vi "read byte array.vi"(9 "specs":T1[](array[typedef]), 10 "elements":T4[](array[typedef]), 11 "byte array":u8[](array[numeric])) -> (0 "error out":errorcluster, 3 "message":variant)   [LabVIEW 2013, in "protocol buffers encoder.lvlib"]
uses:
  protocol buffers encoder.lvlib
  semiparse.ctl
  wire type.ctl
  message specification.ctl
  field descriptor.ctl
  quantity.ctl
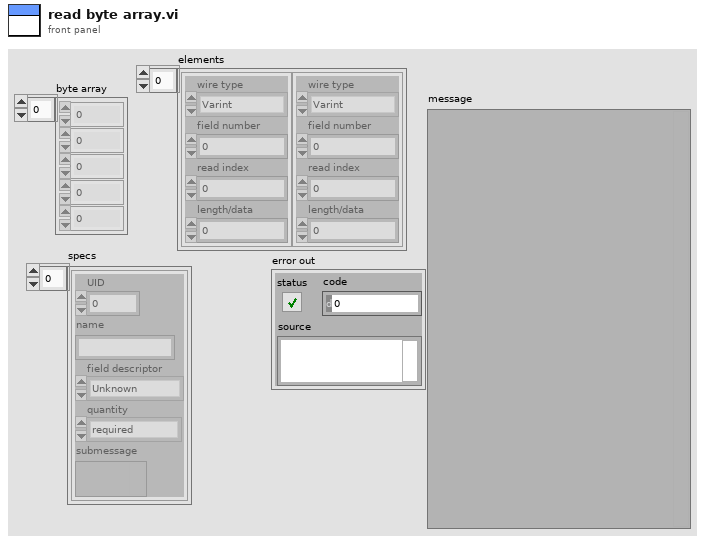
[diagram p1: front panel]
types:
  T1 = typedef "protocol buffers encoder.lvlib/message specification.ctl" = cluster{"UID":u64, "name":string, "field descriptor":T2, "quantity":T3, "submessage":variant}
  T2 = typedef "protocol buffers encoder.lvlib/field descriptor.ctl" = enum16{"Unknown", "dbl", "sgl", "i64", "u64", "i32", "fixed64", "fixed32", "bool", "string", "group", "message", "bytes", "u32", "enum", "sfixed32", "sfixed64", "sint32", "sint64"}
  T3 = typedef "protocol buffers encoder.lvlib/quantity.ctl" = enum16{"required", "optional", "repeated", "repeated/packed"}
  T4 = typedef "protocol buffers encoder.lvlib/semiparse.ctl" = cluster{"wire type":T5, "field number":u64, "read index":i32, "length/data":u64}
  T5 = typedef "protocol buffers encoder.lvlib/wire type.ctl" = enum8{"Varint", "64 bit", "Length Delimited", "Start Group", "End Group", "32 bit"}
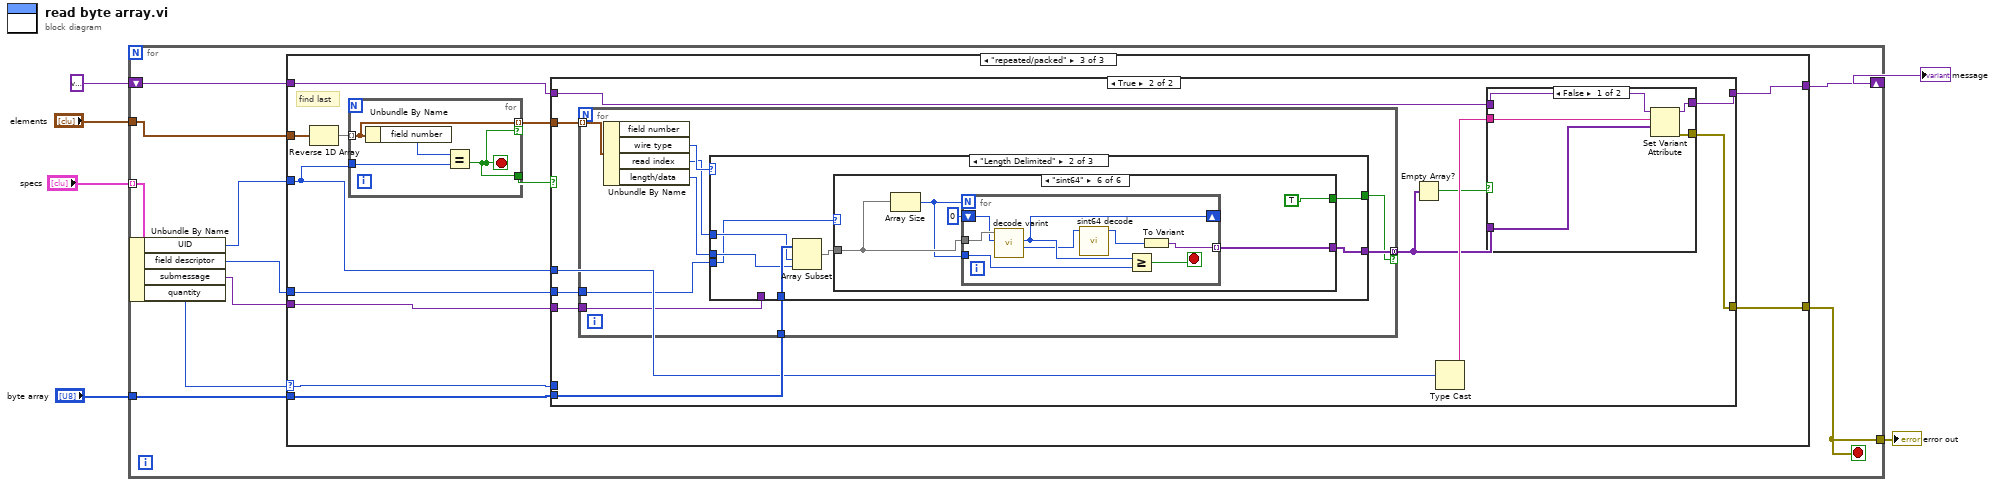
[diagram p0: block diagram]
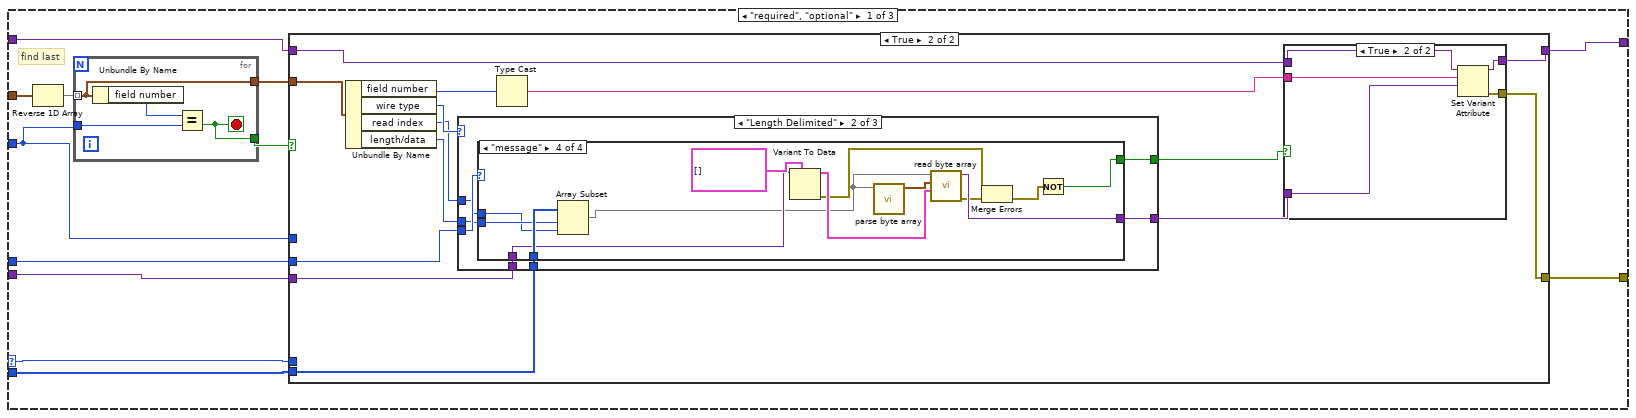
[diagram p2: hidden frame]
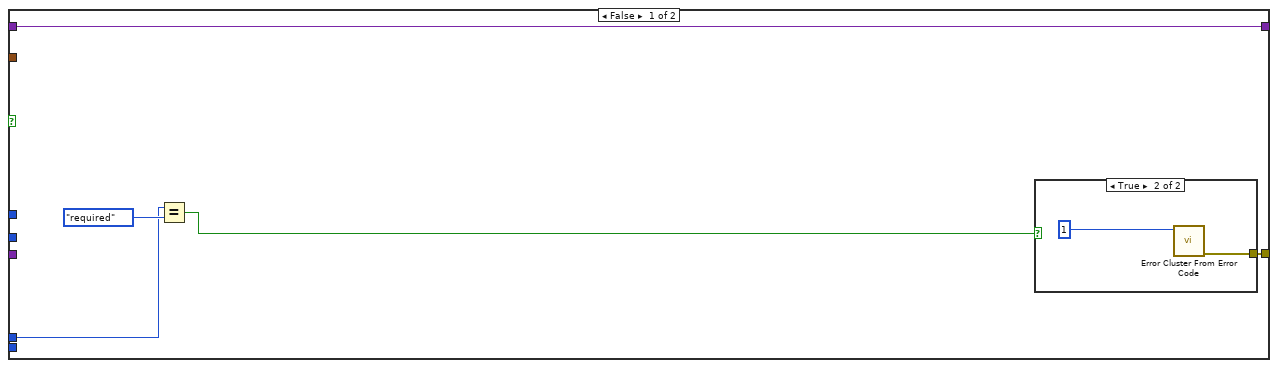
[diagram p3: hidden frame]
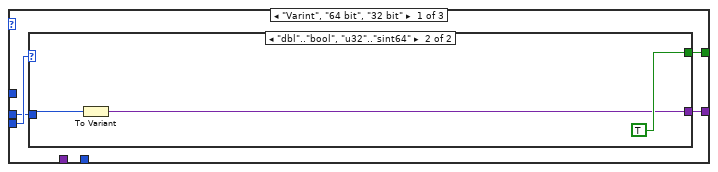
[diagram p5: hidden frame]
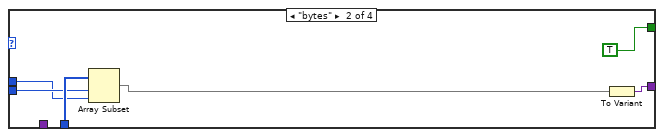
[diagram p8: hidden frame]
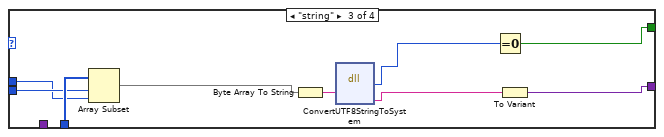
[diagram p9: hidden frame]
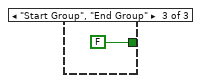
[diagram p10: hidden frame]
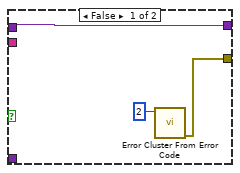
[diagram p11: hidden frame]
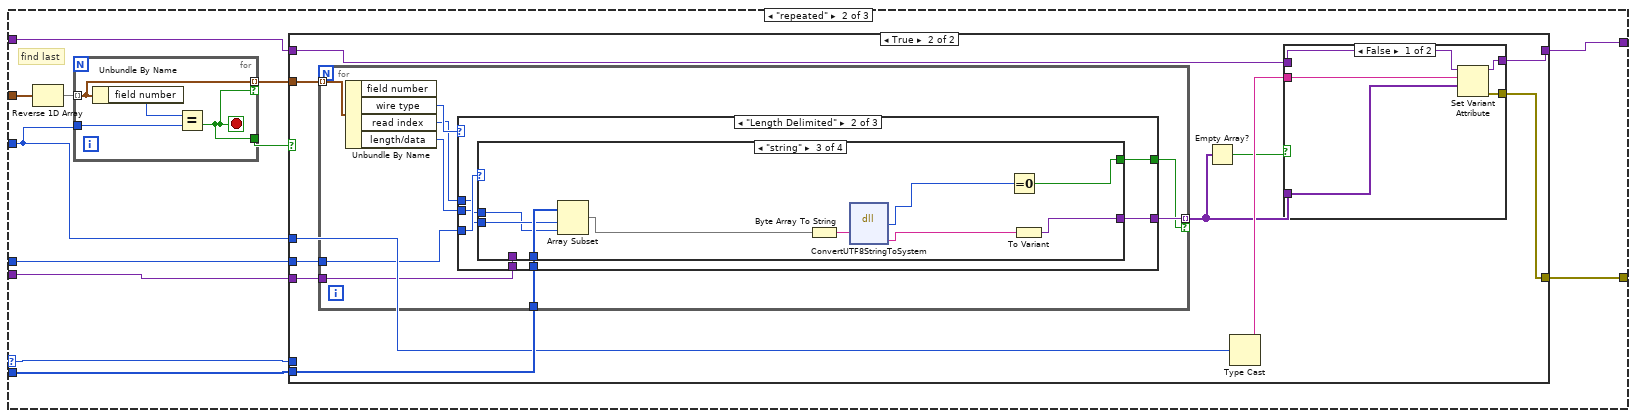
[diagram p12: hidden frame]
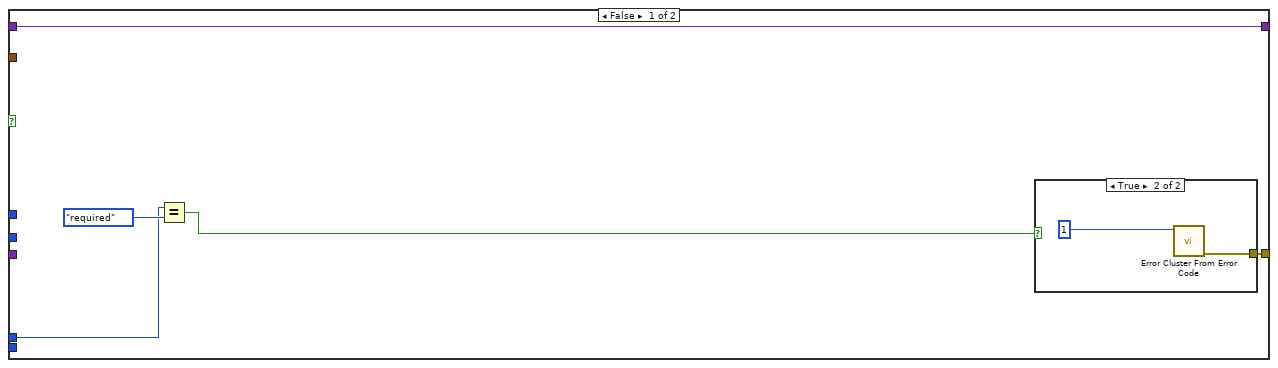
[diagram p13: hidden frame]
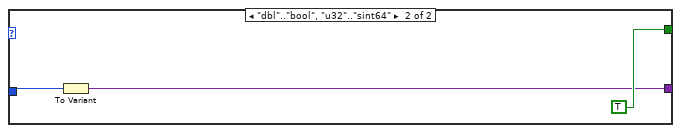
[diagram p16: hidden frame]
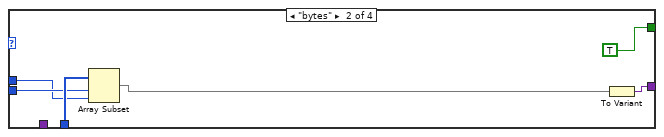
[diagram p18: hidden frame]
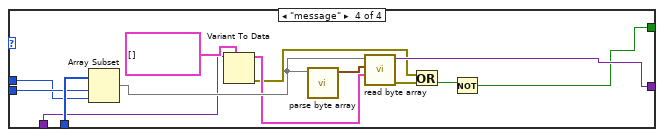
[diagram p19: hidden frame]
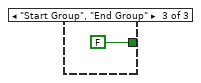
[diagram p20: hidden frame]
diagram:
  n1 = for {
    tunnel: "elements" -> [w12]
    shift-right: [w11] -> w4
    shift-left: variant ("message") -> [w14]
    tunnel: "byte array" -> [w7]
    tunnel: "specs" -> [w16] mode=indexing
    tunnel: [w8] -> w1
    stop <- w8 stop-if-true
    n2 = Unbundle By Name(w16) -> ("UID"=w13:u64, "field descriptor"=w10:T2, "submessage"=w9:variant, "quantity"=w15:T3)
    n3 = case shown="\"repeated/packed\"" w15 {
      selector: w15 -> [w25 w113 w207]
      tunnel: w14 -> [w23 w111 w205]
      tunnel: w13 -> [w21 w109 w203]
      tunnel: w12 -> [w28 w116 w210]
      tunnel: [w24 w112 w206] -> w11
      tunnel: w10 -> [w20 w108 w202]
      tunnel: w9 -> [w19 w107 w201]
      tunnel: [w18 w106 w200] -> w8
      tunnel: w7 -> [w17 w105 w199]
      frame "required", "optional" {
        # "find last"
        n4 = Reverse 1D Array(array=w28) -> (reversed array=w27:T4[])
        n5 = for {
          tunnel: w27 -> [w102] mode=indexing
          tunnel: w21 -> [w103]
          tunnel: [w102] -> w22
          tunnel: [w101] -> w26
          stop <- w101 stop-if-true
          n6 = Unbundle By Name(w102) -> ("field number"=w104:u64)
          n7 = Equal?(x=w104, y=w103) -> (x = y?=w101:bool)
        }
        n8 = case shown="True" w26 {
          tunnel: w25 -> [w32 _]
          tunnel: [w31 w49] -> w24
          tunnel: w23 -> [w31 w48]
          tunnel: w22 -> [_ w47]
          tunnel: w21 -> [_ _]
          tunnel: w20 -> [_ w41]
          tunnel: w19 -> [_ w36]
          tunnel: [w29 w44] -> w18
          tunnel: w17 -> [_ w37]
          frame False {
            n9 = Equal?(x=w32, y=quantity."required") -> (x = y?=w30:bool)
            n10 = case shown="True" w30 {
              tunnel: [_ w35] -> w29
              frame False {
              }
              frame True {
                n11 = call <vilib>:"Error Cluster From Error Code.vi"("error code (0)"=1) -> ("error out"=w35:errorcluster)  [unwired: 8 in]
              }
            }
          }
          frame True {
            n12 = Unbundle By Name(w47) -> ("field number"=w46:u64, "wire type"=w43:T5, "read index"=w40:i32, "length/data"=w39:u64)
            n13 = case shown="\"Length Delimited\"" w43 {
              tunnel: [w52 w62 FALSE] -> w42
              tunnel: w41 -> [w53 w63 _]
              tunnel: w40 -> [_ w60 _]
              tunnel: w39 -> [w51 w59 _]
              tunnel: [w50 w57 _] -> w38
              tunnel: w37 -> [_ w61 _]
              tunnel: w36 -> [_ w58 _]
              frame "Varint", "64 bit", "32 bit" {
                n14 = case shown="\"dbl\"..\"bool\", \"u32\"..\"sint64\"" w53 {
                  tunnel: [_ TRUE] -> w52
                  tunnel: w51 -> [_ w55]
                  tunnel: [_ w54] -> w50
                  frame "Unknown", Default {
                  }
                  frame "dbl".."bool", "u32".."sint64" {
                    n15 = To Variant(anything=w55) -> (Variant=w54:variant)
                  }
                }
              }
              frame "Length Delimited" {
                n16 = case shown="\"message\"" w63 {
                  tunnel: [_ TRUE w70 w81] -> w62
                  tunnel: w61 -> [_ w68 w78 w91]
                  tunnel: w60 -> [_ w67 w77 w90]
                  tunnel: w59 -> [_ w66 w76 w89]
                  tunnel: w58 -> [_ _ _ w86]
                  tunnel: [_ w64 w75 w83] -> w57
                  frame "Unknown", Default {
                  }
                  frame "bytes" {
                    n17 = Array Subset(array=w68, index=w67, length=w66) -> (w65:u8[])
                    n18 = To Variant(anything=w65) -> (Variant=w64:variant)
                  }
                  frame "string" {
                    n19 = Array Subset(array=w78, index=w77, length=w76) -> (w73:u8[])
                    n20 = Byte Array To String(unsigned byte array=w73) -> (string=w74:string)
                    n21 = dll-call lib="LabVIEW" fn="ConvertUTF8StringToSystem"("input"=w74) -> ("mgerr"=w72:i32, "output"=w71:string)  [unwired: 5 in, 2 out]
                    n22 = Equal To 0?(x=w72) -> (x = 0?=w70:bool)
                    n23 = To Variant(anything=w71) -> (Variant=w75:variant)
                  }
                  frame "message" {
                    n24 = Array Subset(array=w91, index=w90, length=w89) -> (w84:u8[])
                    n25 = Variant To Data(type=T1[] [] ("specs"), Variant=w86) -> (data=w85:T1[], error out=w79:errorcluster)  [unwired: 1 in]
                    n26 = call "parse byte array.vi"("byte array"=w84) -> ("elements"=w87:T4[])  [unwired: 10 in]
                    n27 = call "read byte array.vi"("specs"=w85, "elements"=w87, "byte array"=w84) -> ("error out"=w82:errorcluster, "message"=w83:variant)  [unwired: 7 in]
                    n28 = Merge Errors(w79, w82) -> (w80:errorcluster)
                    n29 = Not(x=w80) -> (.not. x?=w81:bool)
                  }
                }
              }
              frame "Start Group", "End Group" {
              }
            }
            n30 = Type Cast(x=w46) -> (*(type *) &x=w45:string)  [unwired: 1 in]
            n31 = case shown="True" w42 {
              tunnel: [w93 w100] -> w49
              tunnel: w48 -> [w93 w99]
              tunnel: w45 -> [_ w98]
              tunnel: [w94 w97] -> w44
              tunnel: w38 -> [_ w96]
              frame False {
                n32 = call <vilib>:"Error Cluster From Error Code.vi"("error code (0)"=2) -> ("error out"=w94:errorcluster)  [unwired: 8 in]
              }
              frame True {
                n33 = Set Variant Attribute(Variant=w99, name=w98, value=w96) -> (Variant out=w100:variant, error out=w97:errorcluster)  [unwired: 1 in, 1 out]
              }
            }
          }
        }
      }
      frame "repeated" {
        # "find last"
        n34 = Reverse 1D Array(array=w116) -> (reversed array=w115:T4[])
        n35 = for {
          tunnel: w115 -> [w196] mode=indexing
          tunnel: w109 -> [w197]
          tunnel: [w196] -> w110 mode=indexing if=w195
          tunnel: [w195] -> w114
          stop <- w195 stop-if-true
          n36 = Unbundle By Name(w196) -> ("field number"=w198:u64)
          n37 = Equal?(x=w198, y=w197) -> (x = y?=w195:bool)
        }
        n38 = case shown="True" w114 {
          tunnel: w113 -> [w120 _]
          tunnel: [w119 w134] -> w112
          tunnel: w111 -> [w119 w133]
          tunnel: w110 -> [_ w132]
          tunnel: w109 -> [_ w126]
          tunnel: w108 -> [_ w129]
          tunnel: w107 -> [_ w127]
          tunnel: [w117 w130] -> w106
          tunnel: w105 -> [_ w128]
          frame False {
            n39 = Equal?(x=w120, y=quantity."required") -> (x = y?=w118:bool)
            n40 = case shown="True" w118 {
              tunnel: [_ w123] -> w117
              frame False {
              }
              frame True {
                n41 = call <vilib>:"Error Cluster From Error Code.vi"("error code (0)"=1) -> ("error out"=w123:errorcluster)  [unwired: 8 in]
              }
            }
          }
          frame True {
            n42 = for {
              tunnel: w132 -> [w143] mode=indexing
              tunnel: w129 -> [w141]
              tunnel: [w138] -> w125 mode=indexing if=w135
              tunnel: w128 -> [w137]
              tunnel: w127 -> [w136]
              n43 = Unbundle By Name(w143) -> ("wire type"=w142:T5, "read index"=w140:i32, "length/data"=w139:u64)  [unwired: 1 out]
              n44 = case shown="\"Length Delimited\"" w142 {
                tunnel: [w146 w156 FALSE] -> w135
                tunnel: w141 -> [w147 w157 _]
                tunnel: w140 -> [_ w154 _]
                tunnel: w139 -> [w145 w153 _]
                tunnel: [w144 w151 _] -> w138
                tunnel: w137 -> [_ w155 _]
                tunnel: w136 -> [_ w152 _]
                frame "Varint", "64 bit", "32 bit" {
                  n45 = case shown="\"Unknown\", Default" w147 {
                    tunnel: [_ TRUE] -> w146
                    tunnel: w145 -> [_ w149]
                    tunnel: [_ w148] -> w144
                    frame "Unknown", Default {
                    }
                    frame "dbl".."bool", "u32".."sint64" {
                      n46 = To Variant(anything=w149) -> (Variant=w148:variant)
                    }
                  }
                }
                frame "Length Delimited" {
                  n47 = case shown="\"string\"" w157 {
                    tunnel: [_ TRUE w164 w175] -> w156
                    tunnel: w155 -> [_ w162 w172 w185]
                    tunnel: w154 -> [_ w161 w171 w184]
                    tunnel: w153 -> [_ w160 w170 w183]
                    tunnel: w152 -> [_ _ _ w178]
                    tunnel: [_ w158 w165 w182] -> w151
                    frame "Unknown", Default {
                    }
                    frame "bytes" {
                      n48 = Array Subset(array=w162, index=w161, length=w160) -> (w159:u8[])
                      n49 = To Variant(anything=w159) -> (Variant=w158:variant)
                    }
                    frame "string" {
                      n50 = Array Subset(array=w172, index=w171, length=w170) -> (w166:u8[])
                      n51 = Byte Array To String(unsigned byte array=w166) -> (string=w169:string)
                      n52 = dll-call lib="LabVIEW" fn="ConvertUTF8StringToSystem"("input"=w169) -> ("mgerr"=w168:i32, "output"=w167:string)  [unwired: 5 in, 2 out]
                      n53 = Equal To 0?(x=w168) -> (x = 0?=w164:bool)
                      n54 = To Variant(anything=w167) -> (Variant=w165:variant)
                    }
                    frame "message" {
                      n55 = Array Subset(array=w185, index=w184, length=w183) -> (w180:u8[])
                      n56 = Variant To Data(type=T1[] [] ("specs"), Variant=w178) -> (data=w177:T1[], error out=w173:errorcluster)  [unwired: 1 in]
                      n57 = call "parse byte array.vi"("byte array"=w180) -> ("elements"=w181:T4[])  [unwired: 10 in]
                      n58 = call "read byte array.vi"("specs"=w177, "elements"=w181, "byte array"=w180) -> ("error out"=w176:errorcluster, "message"=w182:variant)  [unwired: 7 in]
                      n59 = Or(x=w173, y=w176) -> (x .or. y?=w174:bool)
                      n60 = Not(x=w174) -> (.not. x?=w175:bool)
                    }
                  }
                }
                frame "Start Group", "End Group" {
                }
              }
            }
            n61 = Empty Array?(array=w125) -> (empty?=w124:bool)
            n62 = Type Cast(x=w126) -> (*(type *) &x=w131:string)  [unwired: 1 in]
            n63 = case shown="False" w124 {
              tunnel: [w191 w192] -> w134
              tunnel: w133 -> [w190 w192]
              tunnel: w131 -> [w189 _]
              tunnel: [w188 w193] -> w130
              tunnel: w125 -> [w187 _]
              frame False {
                n64 = Set Variant Attribute(Variant=w190, name=w189, value=w187) -> (Variant out=w191:variant, error out=w188:errorcluster)  [unwired: 1 in, 1 out]
              }
              frame True {
                n65 = call <vilib>:"Error Cluster From Error Code.vi"("error code (0)"=2) -> ("error out"=w193:errorcluster)  [unwired: 8 in]
              }
            }
          }
        }
      }
      frame "repeated/packed" {
        # "find last"
        n66 = Reverse 1D Array(array=w210) -> (reversed array=w209:T4[])
        n67 = for {
          tunnel: w209 -> [w308] mode=indexing
          tunnel: w203 -> [w309]
          tunnel: [w308] -> w204 mode=indexing if=w307
          tunnel: [w307] -> w208
          stop <- w307 stop-if-true
          n68 = Unbundle By Name(w308) -> ("field number"=w310:u64)
          n69 = Equal?(x=w310, y=w309) -> (x = y?=w307:bool)
        }
        n70 = case shown="True" w208 {
          tunnel: w207 -> [w214 _]
          tunnel: [w213 w228] -> w206
          tunnel: w205 -> [w213 w227]
          tunnel: w204 -> [_ w226]
          tunnel: w203 -> [_ w220]
          tunnel: w202 -> [_ w223]
          tunnel: w201 -> [_ w221]
          tunnel: [w211 w224] -> w200
          tunnel: w199 -> [_ w222]
          frame False {
            n71 = Equal?(x=w214, y=quantity."required") -> (x = y?=w212:bool)
            n72 = case shown="True" w212 {
              tunnel: [_ w217] -> w211
              frame False {
              }
              frame True {
                n73 = call <vilib>:"Error Cluster From Error Code.vi"("error code (0)"=1) -> ("error out"=w217:errorcluster)  [unwired: 8 in]
              }
            }
          }
          frame True {
            n74 = for {
              tunnel: w226 -> [w237] mode=indexing
              tunnel: w223 -> [w235]
              tunnel: [w232] -> w219 mode=concatenating if=w229
              tunnel: w222 -> [w231]
              tunnel: w221 -> [w230]
              n75 = Unbundle By Name(w237) -> ("wire type"=w236:T5, "read index"=w234:i32, "length/data"=w233:u64)  [unwired: 1 out]
              n76 = case shown="\"Length Delimited\"" w236 {
                tunnel: [FALSE w240 FALSE] -> w229
                tunnel: w235 -> [_ w242 _]
                tunnel: w234 -> [_ w244 _]
                tunnel: w233 -> [_ w243 _]
                tunnel: [_ w239 _] -> w232
                tunnel: w231 -> [_ w245 _]
                tunnel: w230 -> [_ _ _]
                frame "Varint", "64 bit", "32 bit" {
                }
                frame "Length Delimited" {
                  n77 = Array Subset(array=w245, index=w244, length=w243) -> (w241:u8[])
                  n78 = case shown="\"sint64\"" w242 {
                    tunnel: [_ TRUE TRUE TRUE TRUE TRUE] -> w240
                    tunnel: w241 -> [_ w249 w256 w261 w273 w286]
                    tunnel: [_ w246 w253 w262 w274 w287] -> w239
                    frame "Unknown", Default {
                    }
                    frame "dbl", "fixed64", "sfixed64" {
                      n79 = Type Cast(type=u64[] [], x=w249) -> (*(type *) &x=w247:u64[])
                      n80 = for {
                        tunnel: w247 -> [w252] mode=indexing
                        tunnel: [w251] -> w246 mode=indexing
                        n81 = To Variant(anything=w252) -> (Variant=w251:variant)
                      }
                    }
                    frame "sgl", "fixed32", "sfixed32" {
                      n82 = Type Cast(type=u32[] [], x=w256) -> (*(type *) &x=w254:u32[])
                      n83 = for {
                        tunnel: w254 -> [w259] mode=indexing
                        tunnel: [w258] -> w253 mode=indexing
                        n84 = To Variant(anything=w259) -> (Variant=w258:variant)
                      }
                    }
                    frame "i64".."i32", "bool", "u32", "enum" {
                      n85 = Array Size(array=w261) -> (size(s)=w260:i32)
                      n86 = for {
                        N: w260 -> [_]
                        shift-right: [w267] -> _
                        shift-left: 0 -> [w270]
                        tunnel: w261 -> [w271]
                        tunnel: [w268] -> w262 mode=indexing
                        tunnel: w260 -> [w266]
                        stop <- w265 stop-if-true
                        n87 = call "decode varint.vi"("read index in"=w270, "byte array in"=w271) -> ("value"=w269:u64, "read index out"=w267:i32)  [unwired: 8 in]
                        n88 = Greater Or Equal?(x=w267, y=w266) -> (x >= y?=w265:bool)
                        n89 = To Variant(anything=w269) -> (Variant=w268:variant)
                      }
                    }
                    frame "sint32" {
                      n90 = Array Size(array=w273) -> (size(s)=w272:i32)
                      n91 = for {
                        N: w272 -> [_]
                        shift-right: [w281] -> _
                        shift-left: 0 -> [w283]
                        tunnel: w273 -> [w284]
                        tunnel: [w282] -> w274 mode=indexing
                        tunnel: w272 -> [w280]
                        stop <- w279 stop-if-true
                        n92 = call "decode varint.vi"("read index in"=w283, "byte array in"=w284) -> ("value"=w278:u64, "read index out"=w281:i32)  [unwired: 8 in]
                        n93 = call "sint32 decode.vi"("zigzag32"=w278) -> ("sint32"=w277:i32)  [unwired: 10 in]
                        n94 = Greater Or Equal?(x=w281, y=w280) -> (x >= y?=w279:bool)
                        n95 = To Variant(anything=w277) -> (Variant=w282:variant)
                      }
                    }
                    frame "sint64" {
                      n96 = Array Size(array=w286) -> (size(s)=w285:i32)
                      n97 = for {
                        N: w285 -> [_]
                        shift-right: [w294] -> _
                        shift-left: 0 -> [w296]
                        tunnel: w286 -> [w297]
                        tunnel: [w295] -> w287 mode=indexing
                        tunnel: w285 -> [w293]
                        stop <- w292 stop-if-true
                        n98 = call "decode varint.vi"("read index in"=w296, "byte array in"=w297) -> ("value"=w290:u64, "read index out"=w294:i32)  [unwired: 8 in]
                        n99 = call "sint64 decode.vi"("zigzag64"=w290) -> ("sint64"=w291:i64)  [unwired: 10 in]
                        n100 = Greater Or Equal?(x=w294, y=w293) -> (x >= y?=w292:bool)
                        n101 = To Variant(anything=w291) -> (Variant=w295:variant)
                      }
                    }
                  }
                }
                frame "Start Group", "End Group" {
                }
              }
            }
            n102 = Empty Array?(array=w219) -> (empty?=w218:bool)
            n103 = Type Cast(x=w220) -> (*(type *) &x=w225:string)  [unwired: 1 in]
            n104 = case shown="False" w218 {
              tunnel: [w303 w304] -> w228
              tunnel: w227 -> [w302 w304]
              tunnel: w225 -> [w301 _]
              tunnel: [w300 w305] -> w224
              tunnel: w219 -> [w299 _]
              frame False {
                n105 = Set Variant Attribute(Variant=w302, name=w301, value=w299) -> (Variant out=w303:variant, error out=w300:errorcluster)  [unwired: 1 in, 1 out]
              }
              frame True {
                n106 = call <vilib>:"Error Cluster From Error Code.vi"("error code (0)"=2) -> ("error out"=w305:errorcluster)  [unwired: 8 in]
              }
            }
          }
        }
      }
    }
  }
  "message" <- w4
  "error out" <- w1
